vi "Calculate Temp AVGs Send Temp.vi"(8 "error in":errorcluster, 10 "New Temps":dbl[][](array[numeric]), 11 "Old Temps":dbl[][][](array[numeric])) -> (0 "error out":errorcluster, 3 "Combined Temps":dbl[][][](array[numeric]))   [LabVIEW 2017, in "Akwizycja.lvlib"]
uses:
  Akwizycja.lvlib
panel:
  in  "Cluster avg t":T1
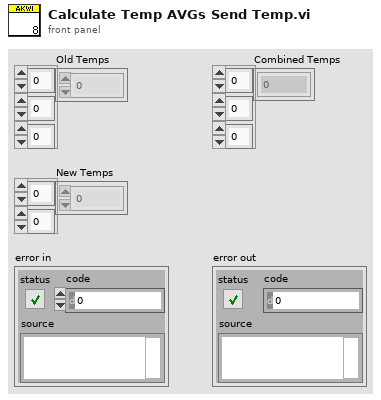
[diagram p1: front panel]
types:
  T1 = cluster{"24h avg":dbl[][], "16h avg":dbl[][], "8h avg":dbl[][], "4h avg":dbl[][], "1h avg":dbl[][]}
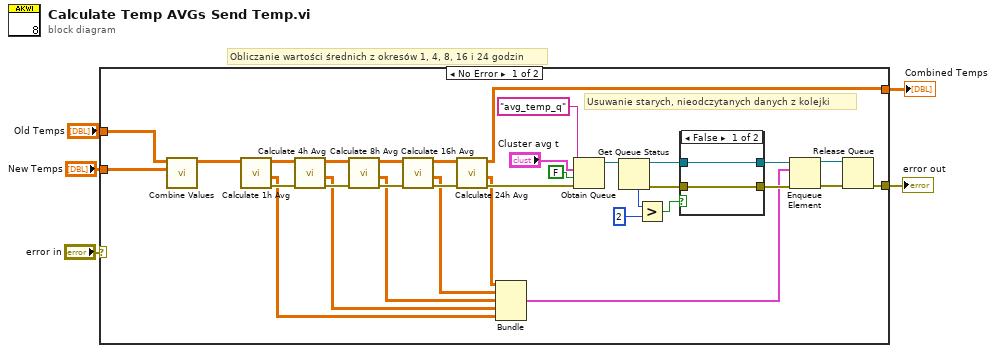
[diagram p0: block diagram]
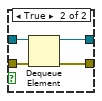
[diagram p2: hidden frame]
diagram:
  # "Obliczanie wartości średnich z okresów 1, 4, 8, 16 i 24 godzin"
  n1 = case shown="No Error" "error in" {
    selector: "error in" -> [_ w46]
    tunnel: "Old Temps" -> [w8 w45]
    tunnel: "New Temps" -> [w7 _]
    tunnel: [w19 w46] -> w3
    tunnel: [w30 w45] -> w2
    frame No Error {
      # "Usuwanie starych, nieodczytanych danych z kolejki"
      n2 = call "Combine Values.vi"("New Values"=w7, "Old Values"=w8) -> ("Combined Values"=w6:dbl[][][])  [unwired: 8 in, 1 out]
      n3 = call "Calculate 1h Avg.vi"("Values in"=w6) -> ("error out"=w31:errorcluster, "1h avg"=w26:dbl[][], "Values out"=w35:dbl[][][])  [unwired: 8 in]
      n4 = call "Calculate 4h Avg.vi"("error in"=w31, "Values in"=w35) -> ("error out"=w32:errorcluster, "4h avg"=w27:dbl[][], "Values out"=w36:dbl[][][])  [unwired: 7 in]
      n5 = call "Calculate 8h Avg.vi"("error in"=w32, "Values in"=w36) -> ("error out"=w33:errorcluster, "8h avg"=w28:dbl[][], "Values out"=w37:dbl[][][])  [unwired: 7 in]
      n6 = call "Calculate 16h Avg.vi"("error in (no error)"=w33, "Values in"=w37) -> ("error out"=w34:errorcluster, "16h avg"=w29:dbl[][], "Values out"=w38:dbl[][][])  [unwired: 7 in]
      n7 = call "Calculate 24h Avg.vi"("error in"=w34, "Values in"=w38) -> ("error out"=w22:errorcluster, "24h avg"=w18:dbl[][], "Values out"=w30:dbl[][][])  [unwired: 7 in]
      n8 = Bundle("24h avg"=w18, "16h avg"=w29, "8h avg"=w28, "4h avg"=w27, "1h avg"=w26) -> (w10:T1)  [unwired: 1 in]
      n9 = Obtain Queue(name (unnamed)="avg_temp_q", element data type="Cluster avg t", create if not found? (T)=FALSE, error in (no error)=w22) -> (queue out=w17:refnum<queue>)  [unwired: 1 in, 2 out]
      n10 = Get Queue Status(queue=w17) -> (queue out=w13:refnum<queue>, error out=w16:errorcluster, # elements in queue=w15:i32)  [unwired: 2 in, 5 out]
      n11 = Greater?(x=w15, y=2) -> (0:w9:bool)
      n12 = case shown="False" w9 {
        tunnel: w16 -> [w39 w44]
        tunnel: w13 -> [w40 w43]
        tunnel: [w40 w42] -> w12
        tunnel: [w39 w41] -> w11
        frame False {
        }
        frame True {
          n13 = Dequeue Element(queue=w43, error in (no error)=w44) -> (queue out=w42:refnum<queue>, error out=w41:errorcluster)  [unwired: 1 in, 2 out]
        }
      }
      n14 = Enqueue Element(queue=w12, element=w10, error in (no error)=w11) -> (queue out=w21:refnum<queue>, error out=w20:errorcluster)  [unwired: 1 in, 1 out]
      n15 = Release Queue(queue=w21, error in (no error)=w20) -> (error out=w19:errorcluster)  [unwired: 1 in, 2 out]
    }
    frame Error {
    }
  }
  "error out" <- w3
  "Combined Temps" <- w2
